vi "19052_rs232_settings.vi"(8 "error in (no error)":errorcluster, 10 "input cluster":T1, 11 "reference in":refnum<visa-resource-name>) -> (0 "error out":errorcluster, 3 "reference out":refnum<visa-resource-name>)   [LabVIEW 2015]
uses:
  Type Definitions/get_visa_resources_data.ctl
  <vilib>/Instr/_visa.llb/VISA Configure Serial Port (Instr).vi
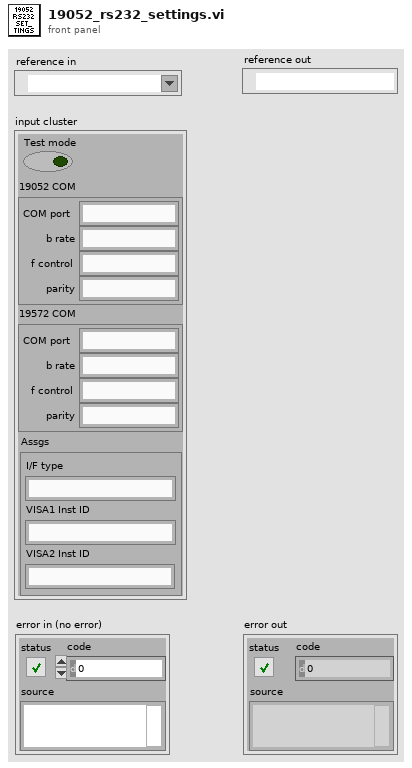
[diagram p1: front panel]
types:
  T1 = typedef "get_visa_resources_data.ctl" = cluster{"Test mode":bool, "19052 COM":cluster{"COM port":string, "b rate":string, "f control":string, "parity":string}, "19572 COM":cluster{"COM port":string, "b rate":string, "f control":string, "parity":string}, "Assgs":cluster{"VISA1 Inst ID":string, "VISA2 Inst ID":string, "I/F type":string}}
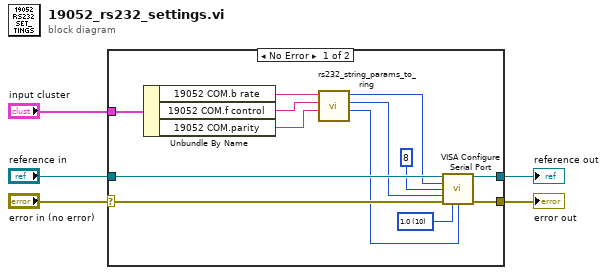
[diagram p0: block diagram]
diagram:
  n1 = case shown="No Error" "error in (no error)" {
    selector: "error in (no error)" -> [w18 w20]
    tunnel: "reference in" -> [w17 w19]
    tunnel: [w9 w19] -> w4
    tunnel: "input cluster" -> [w13 _]
    tunnel: [w10 w20] -> w1
    frame No Error {
      w12 = u16 10 items=["1.0"=10, "1.5"=15, "2.0"=20] ("stop bits (10: 1 bit)")
      n2 = Unbundle By Name(w13) -> ("19052 COM.b rate"=w16:string, "19052 COM.f control"=w15:string, "19052 COM.parity"=w14:string)
      n3 = call "rs232_string_params_to_ring.vi"("flow control string"=w14, "parity string"=w15, "baud rate string"=w16) -> ("Flow control"=w6:u16, "Parity"=w7:enum16{"None", "Odd", "Even", "Mark", "Space"}, "Baud rate"=w8:u32)  [unwired: 6 in]
      n4 = call-poly "VISA Configure Serial Port"("VISA resource name"=w17, "baud rate (9600)"=w8, "data bits (8)"=u16 8, "parity (0:none)"=w7, "error in (no error)"=w18, "stop bits (10: 1 bit)"=w12, "flow control (0:none)"=w6) -> ("VISA resource name out"=w9:refnum<visa-resource-name>, "error out"=w10:errorcluster)  [unwired: 7 in]
    }
    frame Error {
    }
  }
  "reference out" <- w4
  "error out" <- w1
